vi "RT Main.vi"() -> ()   [LabVIEW 2016]
doc: "This template is for the Queued Message Handler design pattern.\n\nThe Event Handling Loop generates messages based on user interface actions.\n\nThe Message Handling Loop processes messages generated by the Event Handling Loop, or by other messages. The messages are string values, so new messages can be added easily to the Message Cases case structure in the Message Handling Loop. Each message cluster can also provide an optional value for Message Data, which is a variant that can be converted to whatever message-specific data is required."
uses:
  Globale Variablen VI/Global Variables.vi
  Globale Variablen VI/AutonomousMode.vi
  Globale Variable/Globale Variable.vi
  <vilib>/FPGAPlugInAG/cRIO-9067/niLvFpga_Open_cRIO-9067.vi
  <vilib>/rvi/interface/common/dynamic/niFpgaDynamicAddResources.vi
  <vilib>/FPGAPlugInAG/Dynamic/niLvFpga_Run_Dynamic.vi
  <vilib>/rvi/interface/nirviOpenFPGA/nirviOpenFPGA.xnode
  FPGA Bitfiles/SUPERFINAL2.5_FPGATarget_CountingFPGA_6pbFvLBtzDM.lvbitx
  FPGA VI/CountingFPGA.vi
  <vilib>/rvi/interface/nirviMethod/nirviMethod.xnode
panel:
  in  "voltage_start":dbl
  in  "starting threshold":dbl
  in  "v_max":dbl
  in  "k_lqr":dbl
  out "error out":errorcluster
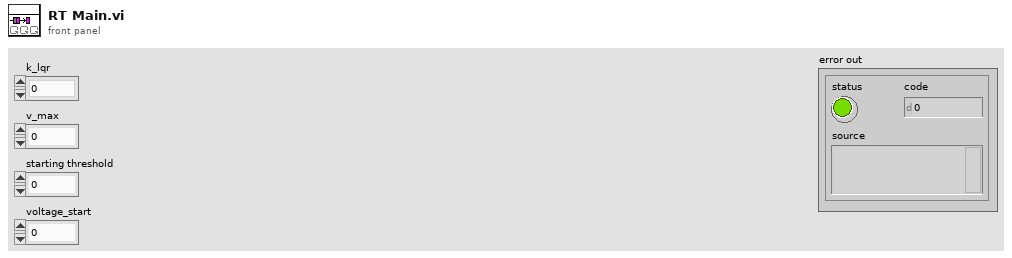
[diagram p1: front panel]
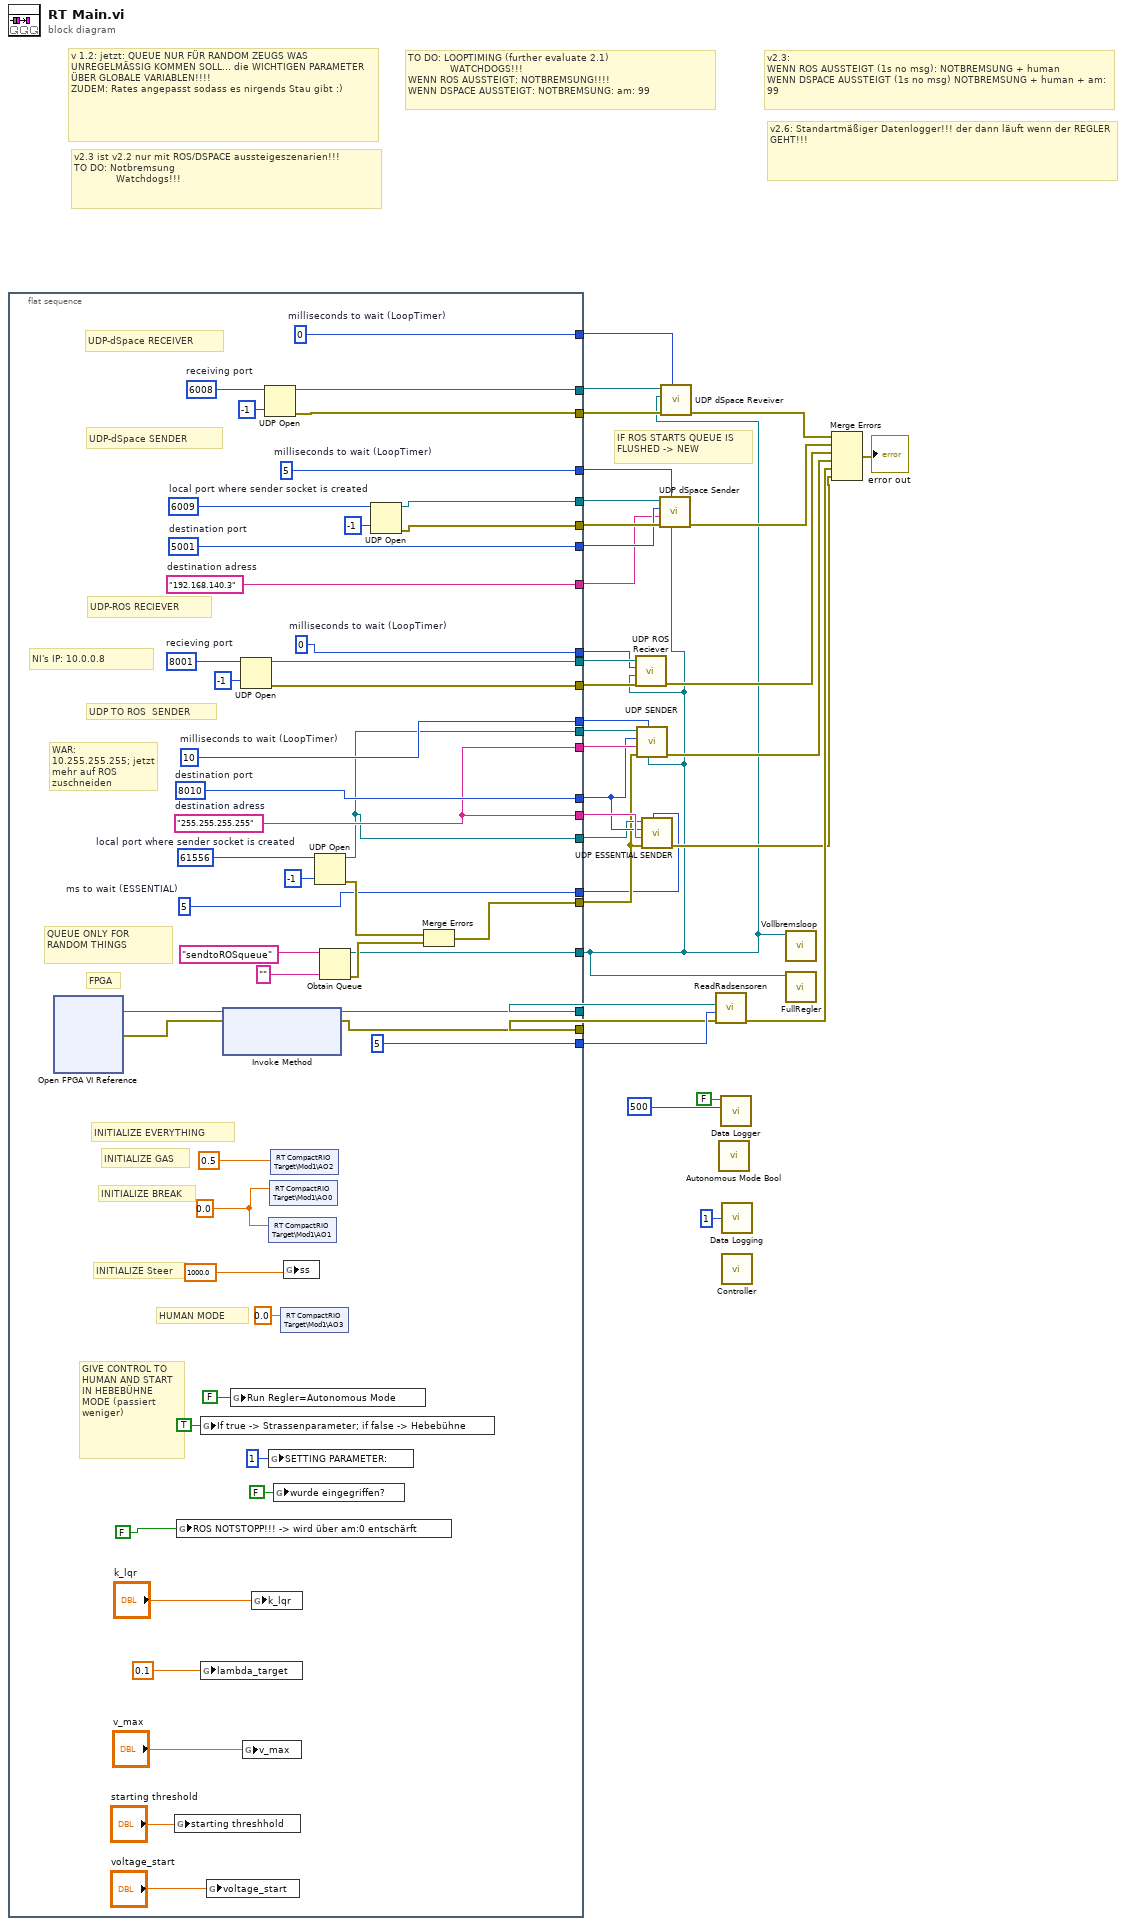
[diagram p0: block diagram]
diagram:
  # "v2.6: Standartmäßiger Datenlogger!!! der dann läuft wenn der REGLER GEHT!!!"
  # "v2.3:\nWENN ROS AUSSTEIGT (1s no msg): NOTBREMSUNG + human\nWENN DSPACE AUSSTEIGT (1s no msg) NOTBREMSUNG + human + am: 99"
  # "TO DO: LOOPTIMING (further evaluate 2.1)\n              WATCHDOGS!!!\nWENN ROS AUSSTEIGT: NOTBREMSUNG!!!!\nWENN DSPACE AUSSTEIGT: NOTBREMSUNG: am: 99"
  # "v2.3 ist v2.2 nur mit ROS/DSPACE aussteigeszenarien!!!\nTO DO: Notbremsung\n              Watchdogs!!!"
  # "IF ROS STARTS QUEUE IS FLUSHED -> NEW"
  # "v 1.2: jetzt: QUEUE NUR FÜR RANDOM ZEUGS WAS UNREGELMÄSSIG KOMMEN SOLL... die WICHTIGEN PARAMETER ÜBER GLOBALE VARIABLEN!!!!\nZUDEM: Rates angepasst sodass es nirgends Stau gibt :)"
  n1 = flat-sequence {
    tunnel: [w73] -> w33
    tunnel: [w72] -> w32
    tunnel: [w71] -> w31
    tunnel: [w70] -> w30
    tunnel: [w69] -> w29
    tunnel: [w68] -> w28
    tunnel: [w67] -> w27
    tunnel: [w66] -> w26
    tunnel: [w45] -> w25
    tunnel: [w60] -> w8
    tunnel: [w65] -> w24
    tunnel: [w64] -> w10
    tunnel: [w46] -> w23
    tunnel: [w63] -> w13
    tunnel: [w59] -> w17
    tunnel: [w58] -> w16
    tunnel: [w57] -> w15
    tunnel: [u32 5 ("milliseconds to wait")] -> w14
    tunnel: [w48] -> w4
    tunnel: [w47] -> w12
    tunnel: [w46] -> w11
    tunnel: [w45] -> w9
    tunnel: [w44] -> w5
    frame #0 {
      w44 = u32 5  # ms to wait (ESSENTIAL)
      w57 = u32 0  # milliseconds to wait (LoopTimer)
      w58 = u32 5  # milliseconds to wait (LoopTimer)
      w59 = u32 0  # milliseconds to wait (LoopTimer)
      w65 = u32 10  # milliseconds to wait (LoopTimer)
      w64 = u16 8010  # destination port
      w76 = u16 61556  # local port where sender socket is created
      w46 = "255.255.255.255"  # destination adress
      w78 = 0.0
      w80 = u16 8001  # recieving port
      w69 = u16 5001  # destination port
      w81 = u16 6009  # local port where sender socket is created
      w68 = "192.168.140.3"  # destination adress
      w82 = u16 6008  # receiving port
      # "HUMAN MODE"
      # "WAR: 10.255.255.255; jetzt mehr auf ROS zuschneiden"
      # "NI's IP: 10.0.0.8"
      # "GIVE CONTROL TO   HUMAN AND START IN HEBEBÜHNE MODE (passiert weniger)"
      # "INITIALIZE EVERYTHING"
      # "QUEUE ONLY FOR RANDOM THINGS"
      # "FPGA"
      # "UDP TO ROS  SENDER"
      # "INITIALIZE Steer"
      # "INITIALIZE BREAK"
      # "INITIALIZE GAS"
      # "UDP-ROS RECIEVER"
      # "UDP-dSpace SENDER"
      # "UDP-dSpace RECEIVER"
      n2 = xnode "Open FPGA VI Reference"() -> ("FPGA VI Reference Out"=w40:refnum<k20>, "error out"=w39:errorcluster)  [unwired: 2 in]
      n3 = global write "Globale Variable.vi" "starting threshhold"("starting threshold") -> ()
      n4 = global write "AutonomousMode.vi" "ROS NOTSTOPP!!! -> wird über am:0 entschärft"(FALSE ("wurde eingegriffen?")) -> ()
      n5 = global write "AutonomousMode.vi" "If true -> Strassenparameter; if false -> Hebebühne"(TRUE ("If true -> Strassenparameter; if false -> Hebebühne")) -> ()
      n6 = global write "Globale Variable.vi" "lambda_target"(0.1 ("lambda_target")) -> ()
      n7 = global write "Globale Variable.vi" "voltage_start"("voltage_start") -> ()
      n8 = xnode "Invoke Method"("FPGA VI Reference In"=w40, "error in"=w39) -> ("FPGA VI Reference Out"=w47:refnum<k20>, "error out"=w63:errorcluster)  [unwired: 1 in]
      n9 = global write "AutonomousMode.vi" "Run Regler=Autonomous Mode"(FALSE ("Autonomous Mode")) -> ()
      n10 = UDP Open(9:-1 ("timeout ms (25000)"), 11:w80) -> (port=w67:refnum<k16>, 0:w66:errorcluster)  [unwired: 3 in, 1 out]
      n11 = global write "Globale Variable.vi" "v_max"("v_max") -> ()
      n12 = global write "Globale Variable.vi" "k_lqr"("k_lqr") -> ()
      n13 = UDP Open(9:-1 ("timeout ms (25000)"), 11:w82) -> (port=w73:refnum<k16>, 0:w72:errorcluster)  [unwired: 3 in, 1 out]
      n14 = shared-variable "RT CompactRIO Target\\Mod1\\AO1"(w78) -> ()  [unwired: 1 in, 1 out]
      n15 = global write "Global Variables.vi" "SETTING PARAMETER:"(1 ("SETTING PARAMETER:\n0: DO NOTHING\n1: SET TO HUMAN MODE\n2: ENABLE REGLER")) -> ()
      n16 = shared-variable "RT CompactRIO Target\\Mod1\\AO0"(w78) -> ()  [unwired: 1 in, 1 out]
      n17 = shared-variable "RT CompactRIO Target\\Mod1\\AO2"(0.5) -> ()  [unwired: 1 in, 1 out]
      n18 = global write "Global Variables.vi" "wurde eingegriffen?"(FALSE ("wurde eingegriffen?")) -> ()
      n19 = shared-variable "RT CompactRIO Target\\Mod1\\AO3"(0.0 ("AO3")) -> ()  [unwired: 1 in, 1 out]
      n20 = global write "Global Variables.vi" "ss"(1000.0 ("ss")) -> ()
      n21 = UDP Open(9:-1 ("timeout ms (25000)"), 11:w76) -> (port=w45:refnum<k16>, 0:w61:errorcluster)  [unwired: 3 in, 1 out]
      n22 = Obtain Queue(name (unnamed)="sendtoROSqueue", element data type="") -> (queue out=w48:refnum<queue>, error out=w62:errorcluster)  [unwired: 3 in, 1 out]
      n23 = UDP Open(9:-1 ("timeout ms (25000)"), 11:w81) -> (port=w71:refnum<k16>, 0:w70:errorcluster)  [unwired: 3 in, 1 out]
      n24 = Merge Errors(w61, w62) -> (w60:errorcluster)
    }
  }
  n25 = call "UDP ROS Reciever.vi"("error in (no error)"=w26, "ENQUE DIRECTLY"=w4, "milliseconds to wait"=w17, "UDP Network Connection in"=w27) -> ("error out"=w20:errorcluster)  [unwired: 7 in]
  n26 = call "UDP SENDER.vi"("queue"=w4, "milliseconds to wait (LoopTimer)"=w24, "error in (no error)"=w8, "destination adress"=w23, "destination port"=w10, "UDP Network Connection in"=w25) -> ("error out"=w19:errorcluster)  [unwired: 5 in]
  n27 = call "UDP ESSENTIAL SENDER.vi"("milliseconds to wait (LoopTimer)"=w5, "error in (no error)"=w8, "destination adress"=w11, "destination port"=w10, "UDP Network Connection in"=w9) -> ("error out"=w6:errorcluster)  [unwired: 6 in]
  n28 = call "UDP dSpace Sender.vi"("ENQUE DIRECTLY"=w4, "milliseconds to wait"=w16, "error in (no error)"=w30, "destination adress"=w28, "destination port"=w29, "UDP Network Connection in"=w31) -> ("error out"=w21:errorcluster)  [unwired: 5 in]
  n29 = call "UDP dSpace Reveiver.vi"("milliseconds to wait"=w15, "error in (no error)"=w32, "ENQUE DIRECTLY"=w4, "UDP Network Connection in"=w33) -> ("error out"=w22:errorcluster)  [unwired: 7 in]
  n30 = call "ReadRadsensoren.vi"("error in (no error)"=w13, "milliseconds to wait"=w14, "FPGA VI Reference Out"=w12) -> ("error out"=w7:errorcluster)  [unwired: 8 in]
  n31 = call "Autonomous Mode Bool.vi"() -> ()  [unwired: 12 in]
  n32 = call "Data Logger.vi"("logging rate (ms)"=u32 500, "YOU WANT TO LOG?"=FALSE) -> ()  [unwired: 10 in]
  n33 = call "Data Logging.vi"("milliseconds to wait"=u32 1) -> ()  [unwired: 1 in]
  n34 = call "Controller.vi"() -> ()  [unwired: 12 in]
  n35 = call "Vollbremsloop.vi"("Queue in"=w4) -> ()  [unwired: 11 in]
  n36 = call "FullRegler.vi"("Queue in"=w4) -> ()  [unwired: 11 in]
  n37 = Merge Errors(w22, w21, w20, w19, w7, w6) -> (→"error out":errorcluster)
